vi "kalman predict step single cycle.vi"(7 "v-feedback":bool, 10 "state in":T1) -> (2 "state out":T1)   [LabVIEW 2010]
uses:
  integrating single axis kalman state.ctl
  <vilib>/rvi/FXPMathLib/FxpInterpret/XNode/nifxpmath_Interpret.xnode
  <vilib>/rvi/FXPMathLib/FxpAdd/XNode/nifxpmath_Add.xnode
  <vilib>/rvi/FXPMathLib/FxpAdd/subVIs/nifxpmath_Add_SimConfig.ctl
  <vilib>/fxp/LVFixedPointQuantizationPolicyTypeDef.ctl
  <vilib>/fxp/LVFixedPointOverflowPolicyTypeDef.ctl
  <vilib>/rvi/FXPMathLib/FxpAdd/simVIs/DllFxpAddTemp_sub.vi
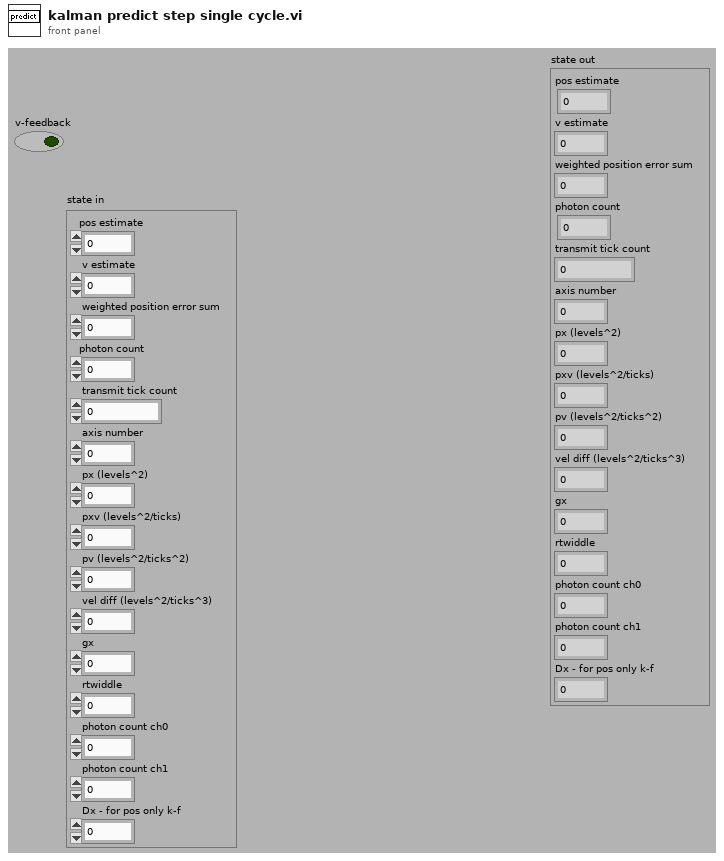
[diagram p1: front panel]
types:
  T1 = typedef "integrating single axis kalman state.ctl" = cluster{"pos estimate":fxp<+/-,32,16>, "v estimate":fxp<+/-,16,0>, "weighted position error sum":fxp<+/-,32,32>, "photon count":u32, "transmit tick count":u32, "axis number":u8, "px (levels^2)":fxp<+,32,19>, "pxv (levels^2/ticks)":fxp<+,32,2>, "pv (levels^2/ticks^2)":fxp<+,32,-14>, "vel diff (levels^2/ticks^3)":fxp<+,24,-22>, "gx":fxp<+,16,8>, "rtwiddle":fxp<+,16,26>, "photon count ch0":u32, "photon count ch1":u32, "Dx - for pos only k-f":fxp<+,32,19>}
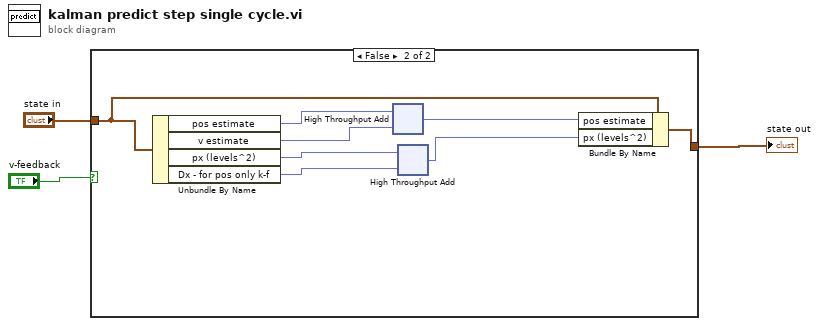
[diagram p0: block diagram]
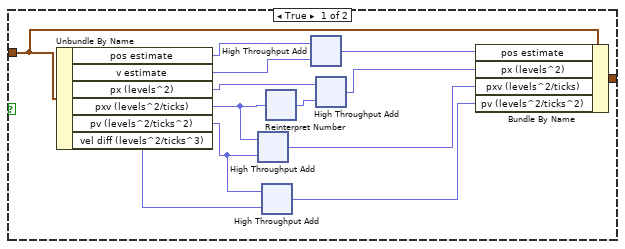
[diagram p2: hidden frame]
diagram:
  n1 = case shown="False" "v-feedback" {
    tunnel: "state in" -> [w10 w147]
    tunnel: [w6 w145] -> w2
    frame True {
      n2 = Unbundle By Name(w10) -> ("pos estimate"=w5:fxp<+/-,32,16>, "v estimate"=w16:fxp<+/-,16,0>, "px (levels^2)"=w15:fxp<+,32,19>, "pxv (levels^2/ticks)"=w13:fxp<+,32,2>, "pv (levels^2/ticks^2)"=w12:fxp<+,32,-14>, "vel diff (levels^2/ticks^3)"=w11:fxp<+,24,-22>)
      n3 = xnode "High Throughput Add"("x"=w13, "y"=w12) -> ("x+y"=w8:fxp<+,32,2>)
      n4 = xnode "High Throughput Add"("x"=w12, "y"=w11) -> ("x+y"=w7:fxp<+,32,-14>)
      n5 = xnode "Reinterpret Number"("x"=w13) -> ("y"=w14:fxp<+,32,3>)
      n6 = xnode "High Throughput Add"("x"=w5, "y"=w16) -> ("x+y"=w4:fxp<+/-,32,16>)
      n7 = xnode "High Throughput Add"("x"=w15, "y"=w14) -> ("x+y"=w9:fxp<+,32,19>)
      n8 = Bundle By Name(cluster=w10, "pos estimate"=w4, "px (levels^2)"=w9, "pxv (levels^2/ticks)"=w8, "pv (levels^2/ticks^2)"=w7) -> (w6:T1)
    }
    frame False {
      n9 = Unbundle By Name(w147) -> ("pos estimate"=w144:fxp<+/-,32,16>, "v estimate"=w149:fxp<+/-,16,0>, "px (levels^2)"=w148:fxp<+,32,19>, "Dx - for pos only k-f"=w142:fxp<+,32,19>)
      n10 = xnode "High Throughput Add"("x"=w144, "y"=w149) -> ("x+y"=w143:fxp<+/-,32,16>)
      n11 = xnode "High Throughput Add"("x"=w148, "y"=w142) -> ("x+y"=w146:fxp<+,32,19>)
      n12 = Bundle By Name(cluster=w147, "pos estimate"=w143, "px (levels^2)"=w146) -> (w145:T1)
    }
  }
  "state out" <- w2
